vi "Ramped Output.vi"(6 "Reinitialize":bool, 9 "Rampup Time":dbl, 11 "Base Power":dbl) -> (3 "Ramped Output":dbl)   [LabVIEW 2013]
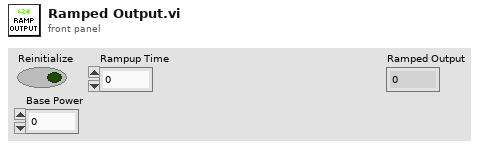
[diagram p1: front panel]
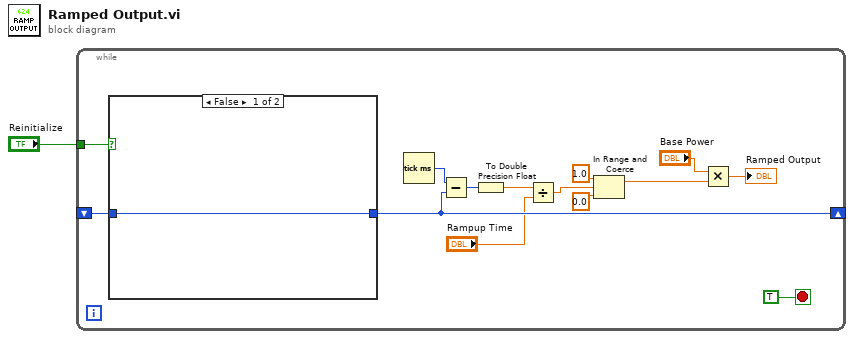
[diagram p0: block diagram]
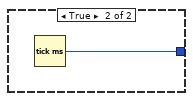
[diagram p2: hidden frame]
diagram:
  n1 = while {
    tunnel: "Reinitialize" -> [w14]
    shift-right: [w11] -> _
    shift-left: _ -> [w13]
    stop <- TRUE stop-if-true
    n2 = case shown="False" w14 {
      tunnel: [w16 w17] -> w11
      tunnel: w13 -> [w16 _]
      frame False {
      }
      frame True {
        n3 = Tick Count (ms)() -> (millisecond timer value=w17:u32)
      }
    }
    n4 = Tick Count (ms)() -> (millisecond timer value=w12:u32)
    n5 = Subtract(x=w12, y=w11) -> (x-y=w10:u32)
    n6 = To Double Precision Float(number=w10) -> (double precision float=w9:dbl)
    n7 = Divide(x=w9, y="Rampup Time") -> (x/y=w2:dbl)
    n8 = In Range and Coerce(upper limit=1.0, x=w2, lower limit=0.0) -> (coerced(x)=w3:dbl)  [unwired: 1 out]
    n9 = Multiply(x="Base Power", y=w3) -> (x*y=→"Ramped Output":dbl)
  }
